vi "GetOneStringFromLIstBox.vi"(11 "ArrayRef in":refnum<vi>) -> (2 "string":string, 3 "ArrayRef out":refnum<vi>)   [LabVIEW 2018, in "Library-Ctrl.lvlib"]
uses:
  Library-Ctrl.lvlib
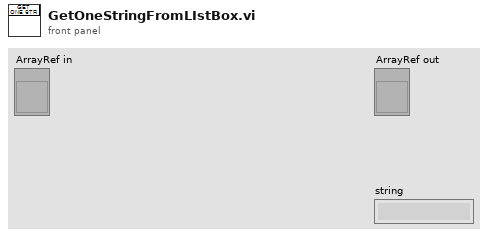
[diagram p1: front panel]
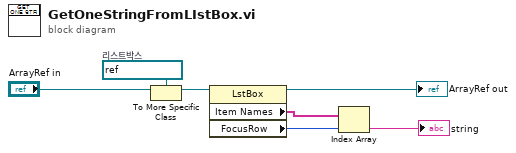
[diagram p0: block diagram]
diagram:
  w3 = refnum<vi> refnum  # 리스트박스
  n1 = To More Specific Class(target class=w3, reference="ArrayRef in") -> (specific class reference=w1:refnum<vi>)  [unwired: 1 in, 1 out]
  n2 = property class="LstBox"(reference=w1) -> (reference out=→"ArrayRef out":refnum<vi>, "Item Names"=w6:string[], "FocusRow"=w5:i32)  [unwired: 1 in, 1 out]
  n3 = Index Array(array=w6, index=w5) -> (element=→"string":string)
